vi "iXonCool.vi"() -> ()   [LabVIEW 2009]
panel:
  out "Detector Y Pixels":i32
  out "Intensity Graph":i32[][](graph)
  in  "Shut Down":bool
  out "Raising Temperature":i32
  in  "Start Acquisition":bool
  out "Return  from Get Acquired Data":u32
  out "Detector X Pixels":i32
  out "Return from GetStatus":u32
  out "Return from Start Acquisition":u32
  out "Cooling":i32
  out "Return from SetTemperature":u32
  in  "Temperature":i32
  out "Return from CheckTimings":u32
  out "Calculated Exposure Value":sgl format="%.2f"
  in  "Exposure Time (secs)":sgl=0.05 format="%.2f"
  out "Return from Initialize":u32
  in  "Trigger":u32(ring) items=["Internal", "External"]
  # "Acquisition Mode: Single Scan\nReadout Mode: Full Vertical Binning\nCools to desired temperature, acquires data and then brings the temperature up to 0 in a controlled way."
  # "Status"
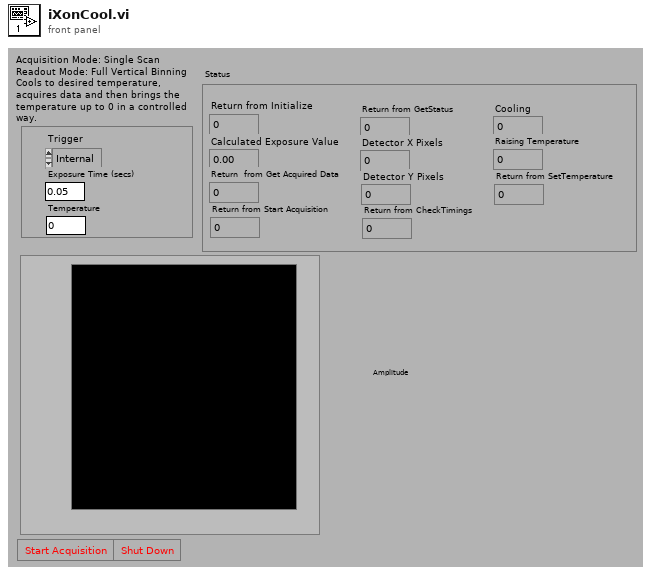
[diagram p1: front panel]
types:
  T1 = typedef "Error Code Enum typedef.ctl" = enum32{"N/A (0)", "DRV_ERROR_CODES", "DRV_SUCCESS", "DRV_VXDNOTINSTALLED", "DRV_ERROR_SCAN", "DRV_ERROR_CHECK_SUM", "DRV_ERROR_FILELOAD", "DRV_UNKNOWN_FUNC", "DRV_ERROR_VXD_INIT", "DRV_ERROR_ADDRESS", "DRV_ERROR_PAGELOCK", "DRV_ERROR_PAGEUNLOCK", "DRV_ERROR_BOARDTEST", "DRV_ERROR_ACK", "DRV_ERROR_UP_FIFO", "DRV_ERROR_PATTERN", "N/A (16)", "DRV_ACQUISITION_ERRORS", "DRV_ACQ_BUFFER", "DRV_ACQ_DOWNFIFO_FULL", "DRV_PROC_UNKONWN_INSTRUCTION", "DRV_ILLEGAL_OP_CODE", "DRV_KINETIC_TIME_NOT_MET", "DRV_ACCUM_TIME_NOT_MET", "DRV_NO_NEW_DATA", "N/A (25)", "DRV_SPOOLERROR", "N/A (27)", "N/A (28)", "N/A (29)", "N/A (30)", "N/A (31)", "N/A (32)", "DRV_TEMPERATURE_CODES", "DRV_TEMPERATURE_OFF", "DRV_TEMPERATURE_NOT_STABILIZED", "DRV_TEMPERATURE_STABILIZED", "DRV_TEMPERATURE_NOT_REACHED", "DRV_TEMPERATURE_OUT_RANGE", "DRV_TEMPERATURE_NOT_SUPPORTED", "DRV_TEMPERATURE_DRIFT", "N/A (41)", "N/A (42)", "N/A (43)", "N/A (44)", "N/A (45)", "N/A (46)", "N/A (47)", "N/A (48)", "DRV_GENERAL_ERRORS", "DRV_INVALID_AUX", "DRV_COF_NOTLOADED", "DRV_FPGAPROG", "DRV_FLEXERROR", "DRV_GPIBERROR", "N/A (55)", "N/A (56)", "N/A (57)", "N/A (58)", "N/A (59)", "N/A (60)", "N/A (61)", "N/A (62)", "N/A (63)", "DRV_DATATYPE", "DRV_DRIVER_ERRORS", "DRV_P1INVALID", "DRV_P2INVALID", "DRV_P3INVALID", "DRV_P4INVALID", "DRV_INIERROR", "DRV_COFERROR", "DRV_ACQUIRING", "DRV_IDLE", "DRV_TEMPCYCLE", "DRV_NOT_INITIALIZED", "DRV_P5INVALID", "DRV_P6INVALID", "DRV_INVALID_MODE", "DRV_INVALID_FILTER", "DRV_I2CERRORS", "DRV_I2CDEVNOTFOUND", "DRV_I2CTIMEOUT", "DRV_P7INVALID", "N/A (84)", "N/A (85)", "N/A (86)", "N/A (87)", "N/A (88)", "N/A (89)", "DRV_IOCERROR", "DRV_VRMVERSIONERROR"}
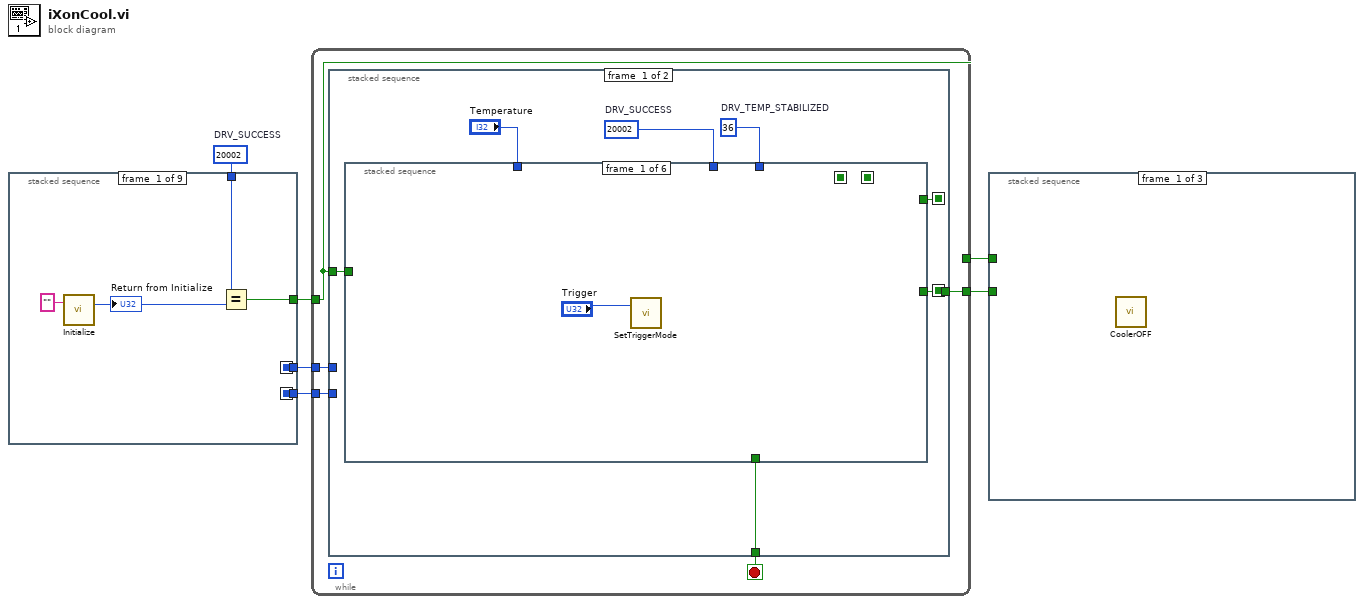
[diagram p0: block diagram]
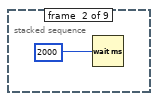
[diagram p2: hidden frame]
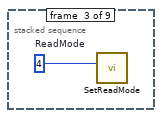
[diagram p3: hidden frame]
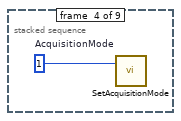
[diagram p4: hidden frame]
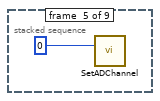
[diagram p5: hidden frame]
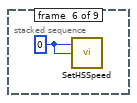
[diagram p6: hidden frame]
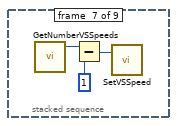
[diagram p7: hidden frame]
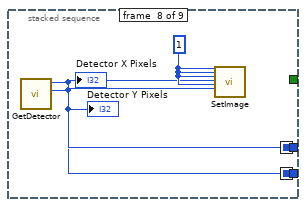
[diagram p8: hidden frame]
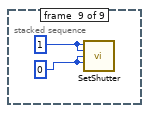
[diagram p9: hidden frame]
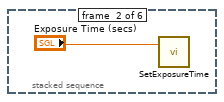
[diagram p10: hidden frame]
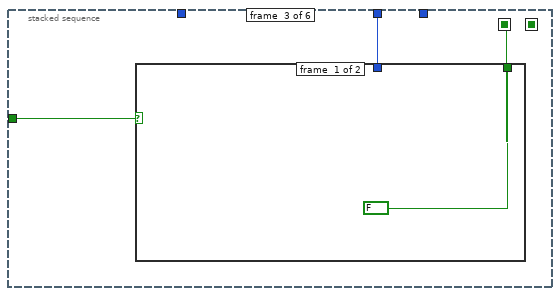
[diagram p11: hidden frame]
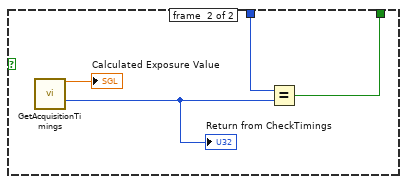
[diagram p12: hidden frame]
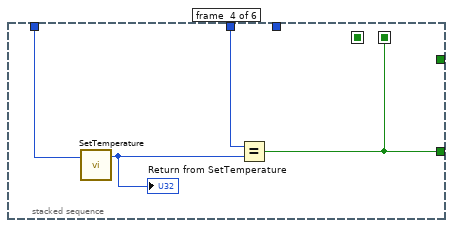
[diagram p13: hidden frame]
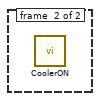
[diagram p15: hidden frame]
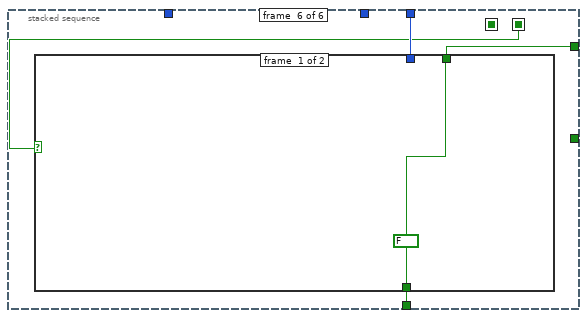
[diagram p16: hidden frame]
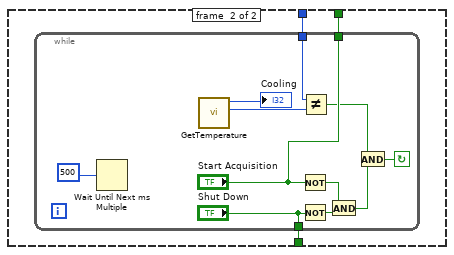
[diagram p17: hidden frame]
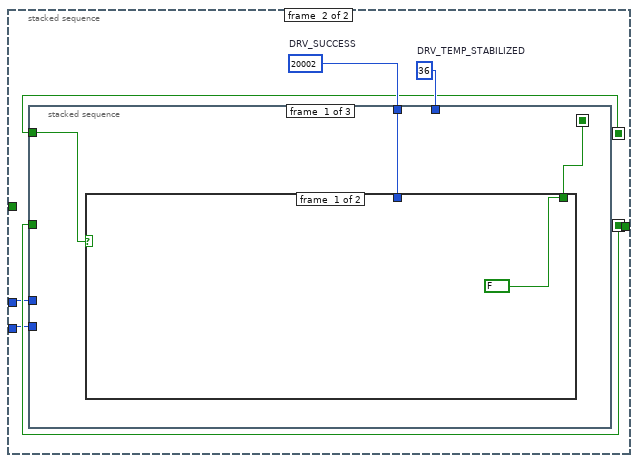
[diagram p18: hidden frame]
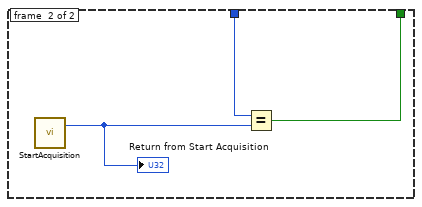
[diagram p19: hidden frame]
diagram:
  w4 = 20002  # DRV_SUCCESS
  n1 = stacked-sequence {
    seq-local: [_ _ _ _ _ _ _ w20 _] -> [_ _ _ _ _ _ _ _ _]
    seq-local: [_ _ _ _ _ _ _ w19 _] -> [_ _ _ _ _ _ _ _ _]
    tunnel: w4 -> [w8 _ _ _ _ _ _ _ _]
    tunnel: [w7 _ _ _ _ _ _ _ _] -> w3
    tunnel: [_ _ _ _ _ _ _ w20 _] -> w2
    tunnel: [_ _ _ _ _ _ _ w19 _] -> w1
    frame #0 {
      n2 = call <userlib>:"Initialize.vi"("directory (\"\")"="" ("directory (\"\")")) -> ("DLL error code"=w10:u32)  [unwired: 1 in, 1 out]
      "Return from Initialize" <- w10
      n3 = Equal?(x=w8, y=w10) -> (x = y?=w7:bool)
    }
    frame #1 {
      n4 = Wait (ms)(milliseconds to wait=u32 2000) -> ()  [unwired: 1 out]
    }
    frame #2 {
      w12 = u16 4  # ReadMode
      n5 = call <userlib>:"SetReadMode.vi"("mode"=w12) -> ()  [unwired: 1 in, 2 out]
    }
    frame #3 {
      w13 = u16 1  # AcquisitionMode
      n6 = call <userlib>:"SetAcquisitionMode.vi"("mode"=w13) -> ()  [unwired: 1 in, 2 out]
    }
    frame #4 {
      n7 = call <userlib>:"SetADChannel.vi"("channel"=0) -> ()  [unwired: 1 in, 2 out]
    }
    frame #5 {
      w15 = 0
      n8 = call <userlib>:"SetHSSpeed.vi"("index"=w15, "type"=w15) -> ()  [unwired: 2 in, 2 out]
    }
    frame #6 {
      n9 = call <userlib>:"GetNumberVSSpeeds.vi"() -> ("number"=w18:i32)  [unwired: 3 in, 2 out]
      n10 = Subtract(x=w18, y=1) -> (x-y=w16:i32)
      n11 = call <userlib>:"SetVSSpeed.vi"("index"=w16) -> ()  [unwired: 1 in, 2 out]
    }
    frame #7 {
      w21 = 1
      n12 = call <userlib>:"GetDetector.vi"() -> ("ypixels"=w20:i32, "xpixels"=w19:i32)  [unwired: 4 in, 2 out]
      "Detector Y Pixels" <- w20
      "Detector X Pixels" <- w19
      n13 = call <userlib>:"SetImage.vi"("hbin"=w21, "vbin"=w21, "hstart"=w21, "hend"=w19, "vstart"=w21, "vend"=w20) -> ()  [unwired: 20 in, 2 out]
    }
    frame #8 {
      w22 = 0
      w23 = 1
      n14 = call <userlib>:"SetShutter.vi"("type"=w23, "mode"=w23, "closingtime"=w22, "openingtime"=w22) -> ()  [unwired: 10 in, 2 out]
    }
  }
  n15 = while {
    tunnel: [w24] -> w6
    tunnel: [w28] -> w5
    tunnel: w3 -> [w24]
    tunnel: w2 -> [w27]
    tunnel: w1 -> [w26]
    stop <- w25 stop-if-true
    n16 = stacked-sequence {
      seq-local: [w35 _] -> [_ w73]
      seq-local: [w34 _] -> [_ w72]
      tunnel: [_ w72] -> w28
      tunnel: w27 -> [_ w71]
      tunnel: w26 -> [_ w70]
      tunnel: [w30 _] -> w25
      tunnel: w24 -> [w29 _]
      frame #0 {
        w31 = 36  # DRV_TEMP_STABILIZED
        w33 = 20002  # DRV_SUCCESS
        n17 = stacked-sequence {
          seq-local: [_ _ w38 _ _ _] -> [_ _ _ _ _ _]
          seq-local: [_ _ _ w46 _ _] -> [_ _ _ _ w50 w53]
          tunnel: w33 -> [_ _ w40 w49 _ _]
          tunnel: "Temperature" -> [_ _ _ w47 _ _]
          tunnel: w31 -> [_ _ _ _ _ w54]
          tunnel: [_ _ _ _ _ w51] -> w35
          tunnel: [_ _ _ w46 _ _] -> w34
          tunnel: [_ _ _ _ _ w52] -> w30
          tunnel: w29 -> [_ _ w39 _ _ _]
          frame #0 {
            n18 = call <userlib>:"SetTriggerMode.vi"("mode"="Trigger") -> ()  [unwired: 1 in, 2 out]
          }
          frame #1 {
            n19 = call <userlib>:"SetExposureTime.vi"("time"="Exposure Time (secs)") -> ()  [unwired: 1 in, 2 out]
          }
          frame #2 {
            n20 = case shown="True" w39 {
              tunnel: w40 -> [_ w43]
              tunnel: [FALSE w45] -> w38
              frame #0 {
              }
              frame #1 {
                n21 = call <userlib>:"GetAcquisitionTimings.vi"() -> ("exposure"=→"Calculated Exposure Value":sgl, "DLL error code"=w42:u32)  [unwired: 11 in, 3 out]
                "Return from CheckTimings" <- w42
                n22 = Equal?(x=w43, y=w42) -> (x = y?=w45:bool)
              }
            }
          }
          frame #3 {
            n23 = call <userlib>:"SetTemperature.vi"("temperature"=w47) -> ("DLL error code"=w48:u32)  [unwired: 1 in, 1 out]
            "Return from SetTemperature" <- w48
            n24 = Equal?(x=w49, y=w48) -> (x = y?=w46:bool)
          }
          frame #4 {
            n25 = case shown="True" w50 {
              frame #0 {
              }
              frame #1 {
                n26 = call <userlib>:"CoolerON.vi"() -> ()  [unwired: 2 in, 2 out]
              }
            }
          }
          frame #5 {
            n27 = case shown="True" w53 {
              tunnel: w54 -> [_ w58]
              tunnel: [w55 w57] -> w52
              tunnel: [w55 w56] -> w51
              frame #0 {
                w55 = FALSE
              }
              frame #1 {
                n28 = while {
                  tunnel: w58 -> [w68]
                  tunnel: ["Shut Down"] -> w57
                  tunnel: ["Start Acquisition"] -> w56
                  stop <- w61 continue-if-true
                  n29 = Wait Until Next ms Multiple(millisecond multiple=u32 500) -> ()  [unwired: 1 out]
                  n30 = call <userlib>:"GetTemperature.vi"() -> ("status"=w66:T1, "temperature"=→"Cooling":i32)  [unwired: 4 in, 2 out]
                  n31 = Not(x="Start Acquisition") -> (.not. x?=w63:bool)
                  n32 = Not(x="Shut Down") -> (.not. x?=w65:bool)
                  n33 = Not Equal?(x=w68, y=w66) -> (x != y?=w60:bool)
                  n34 = And(x=w63, y=w65) -> (x .and. y?=w59:bool)
                  n35 = And(x=w60, y=w59) -> (x .and. y?=w61:bool)
                }
              }
            }
          }
        }
      }
      frame #1 {
        w74 = 36  # DRV_TEMP_STABILIZED
        w75 = 20002  # DRV_SUCCESS
        n36 = stacked-sequence {
          seq-local: [w77 _ _] -> [_ w83 _]
          tunnel: w75 -> [w78 _ _]
          tunnel: w74 -> [_ _ _]
          tunnel: w73 -> [w76 _ _]
          tunnel: w72 -> [_ _ _]
          tunnel: w71 -> [_ _ w89]
          tunnel: w70 -> [_ _ w88]
          frame #0 {
            n37 = case shown="True" w76 {
              tunnel: [FALSE w82] -> w77
              tunnel: w78 -> [_ w81]
              frame #0 {
              }
              frame #1 {
                n38 = call <userlib>:"StartAcquisition.vi"() -> ("DLL error code"=w80:u32)  [unwired: 2 in, 1 out]
                "Return from Start Acquisition" <- w80
                n39 = Equal?(x=w81, y=w80) -> (x = y?=w82:bool)
              }
            }
          }
          frame #1 {
            n40 = case shown="True" w83 {
              frame #0 {
              }
              frame #1 {
                n41 = while {
                  stop <- w86 continue-if-true
                  w85 = u16 72  # DRV ACQUIRING
                  n42 = call <userlib>:"GetStatus.vi"() -> ("status"=w84:T1)  [unwired: 3 in, 2 out]
                  "Return from GetStatus" <- w84
                  n43 = Wait Until Next ms Multiple(millisecond multiple=u32 50) -> ()  [unwired: 1 out]
                  n44 = Equal?(x=w84, y=w85) -> (x = y?=w86:bool)
                }
              }
            }
          }
          frame #2 {
            n45 = Multiply(x=w89, y=w88) -> (x*y=w92:i32)
            n46 = call <userlib>:"GetAcquiredData.vi"("size"=w92) -> ("DLL error code"=→"Return  from Get Acquired Data":u32, "array"=w91:i32[])  [unwired: 2 in, 1 out]
            n47 = Reshape Array(w91, w89, w88) -> (→"Intensity Graph":i32[][])
          }
        }
      }
    }
  }
  n48 = stacked-sequence {
    tunnel: w5 -> [_ w94 _]
    tunnel: w6 -> [_ _ w99]
    frame #0 {
      n49 = call <userlib>:"CoolerOFF.vi"() -> ()  [unwired: 2 in, 2 out]
    }
    frame #1 {
      n50 = case shown="True" w94 {
        frame #0 {
        }
        frame #1 {
          n51 = while {
            stop <- w97 continue-if-true
            n52 = call <userlib>:"GetTemperature.vi"() -> ("temperature"=w96:i32)  [unwired: 4 in, 3 out]
            "Raising Temperature" <- w96
            n53 = Less?(x=w96, y=i16 0) -> (x < y?=w97:bool)
            n54 = Wait Until Next ms Multiple(millisecond multiple=u32 500) -> ()  [unwired: 1 out]
          }
        }
      }
    }
    frame #2 {
      n55 = case shown="True" w99 {
        frame #0 {
        }
        frame #1 {
          n56 = call <userlib>:"ShutDown.vi"() -> ()  [unwired: 2 in, 2 out]
        }
      }
    }
  }
